vi "New Edit Element.vi"(8 "error in (no error)":errorcluster, 11 "Component-A in":refnum<class "Component-A.lvclass">) -> (0 "error out":errorcluster, 3 "Component-A out":refnum<class "Component-A.lvclass">)   [LabVIEW 2018, in "Component-A.lvclass"]
uses:
  Component-A.lvclass
  <vilib>/ErrorRing/Error Ring.xnode
  <vilib>/Utility/error.llb/Error Cluster From Error Code.vi
  U:/modules/labview-orm/demo/Component.lvclass
  U:/modules/labview-orm/_Serializable Base Object/_ISerializable.lvclass
panel:
  out "uid":u64
  in  "active":bool
  in  "RelatedIssues":dbl format="%.5g"
  in  "owner":string
  in  "isEssencial_":bool
  in  "status":u8
  in  "isObsolete":bool
  in  "cancel button":bool
  in  "ok button":bool
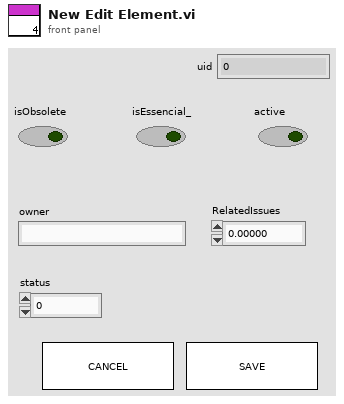
[diagram p1: front panel]
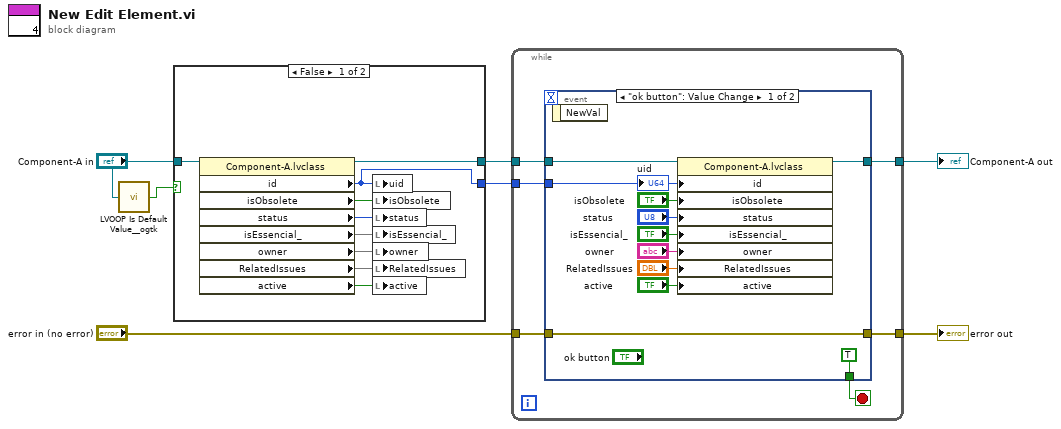
[diagram p0: block diagram]
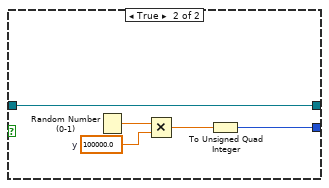
[diagram p2: hidden frame]
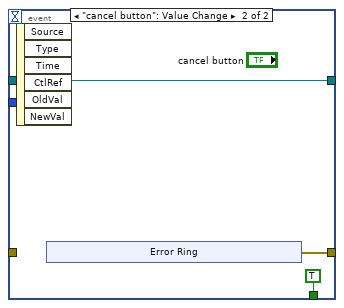
[diagram p3: hidden frame]
diagram:
  n1 = call <userlib>:"LVOOP Is Default Value__ogtk.vi"("Object"="Component-A in") -> ("Is Default Value?"=w2:bool)
  n2 = case shown="False" w2 {
    tunnel: [w14 w18] -> w4
    tunnel: "Component-A in" -> [w16 w17]
    tunnel: [w15 w17] -> w1
    frame False {
      n3 = property class="Component-A.lvclass"(reference=w16) -> (reference out=w15:refnum<class "Component-A.lvclass">, "id"=w14:i32, "isObsolete"=w13:bool, "status"=w12:u8, "isEssencial_"=w11, "owner"=w10, "RelatedIssues"=w9, "active"=w8:bool)  [unwired: 1 in, 1 out]
      n4 = local write "uid"(w14) -> ()
      n5 = local write "isObsolete"(w13) -> ()
      n6 = local write "status"(w12) -> ()
      n7 = local write "isEssencial_"(w11) -> ()
      n8 = local write "owner"(w10) -> ()
      n9 = local write "RelatedIssues"(w9) -> ()
      n10 = local write "active"(w8) -> ()
    }
    frame True {
      w20 = 100000.0  # y
      n11 = Random Number (0-1)() -> (number: 0 to 1=w21:dbl)
      n12 = Multiply(x=w21, y=w20) -> (x*y=w19:dbl)
      n13 = To Unsigned Quad Integer(1:w19) -> (0:w18:u64)
    }
  }
  n14 = while {
    tunnel: "error in (no error)" -> [w24]
    tunnel: w1 -> [w27]
    tunnel: [w26] -> w6
    tunnel: [w25] -> w5
    tunnel: w4 -> [w22]
    stop <- w23 stop-if-true
    n15 = event shown="[0] \"ok button\": Value Change" {
      selector: _ -> [_ _]
      dyn-events: _ -> [_ _]
      timeout: _ -> [_ _]
      tunnel: w27 -> [w38 w41]
      tunnel: [w37 w41] -> w26
      tunnel: [w36 w40] -> w25
      tunnel: w24 -> [w36 _]
      tunnel: [TRUE TRUE] -> w23
      tunnel: w22 -> [w34 _]
      event "ok button": Value Change {
        n16 = event-data() -> ()  [unwired: 1 in, 1 out]
        n17 = property class="Component-A.lvclass"(reference=w38, "id"=w34, "isObsolete"="isObsolete", "status"="status", "isEssencial_"="isEssencial_", "owner"="owner", "RelatedIssues"="RelatedIssues", "active"="active") -> (reference out=w37:refnum<class "Component-A.lvclass">)  [unwired: 1 in, 1 out]
        "uid" <- w34
      }
      event "cancel button": Value Change {
        n18 = event-data() -> ()  [unwired: 1 in, 6 out]
        n19 = xnode "Error Ring"() -> ("error out"=w40:errorcluster)
      }
    }
  }
  "error out" <- w5
  "Component-A out" <- w6
